vi "FilePathGlobal.vi"(0 "Image Path":path, 1 "set?":bool) -> (2 "Image Path 2":path, 3 "substring":string, 4 "stripped path":path)   [LabVIEW 2009]
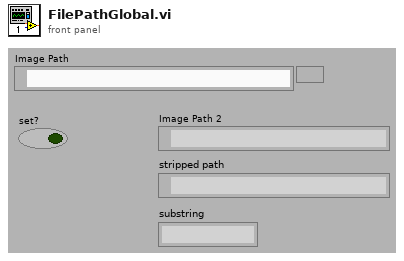
[diagram p1: front panel]
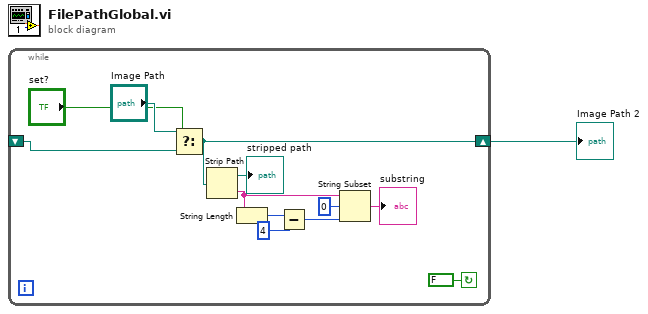
[diagram p0: block diagram]
diagram:
  n1 = while {
    shift-right: [w9] -> w1
    shift-left: _ -> [w12]
    stop <- FALSE continue-if-true
    n2 = Select(t="Image Path", s="set?", f=w12) -> (s? t:f=w9:path)
    n3 = Strip Path(path=w9) -> (stripped path=→"stripped path":path, name=w6:string)
    n4 = String Length(string=w6) -> (length=w8:i32)
    n5 = Subtract(x=w8, y=4) -> (x-y=w3:i32)
    n6 = String Subset(string=w6, offset (0)=0, length (rest)=w3) -> (substring=→"substring":string)
  }
  "Image Path 2" <- w1
